vi "Read Logger.vi"(8 "error in (no error)":errorcluster, 11 "CoreOperation in":refnum<class "CoreOperation.lvclass">) -> (0 "error out":errorcluster, 2 "Logger.lvclass":refnum<class "Logger.lvclass">, 3 "CoreOperation out":refnum<class "CoreOperation.lvclass">)   [LabVIEW 2014, in "CoreOperation.lvclass"]
uses:
  CoreOperation.lvclass
  Utilities/Logger/Logger.lvclass
  CoreOperation.lvclass/CoreOperation.ctl
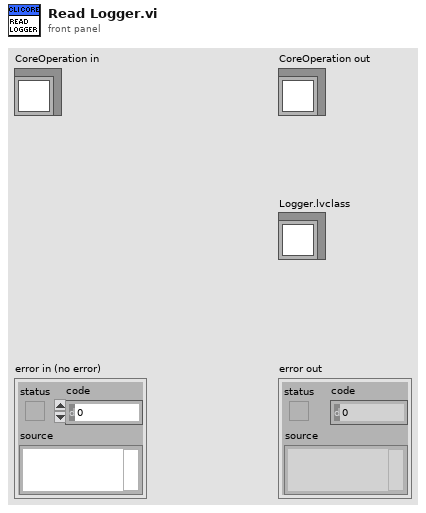
[diagram p1: front panel]
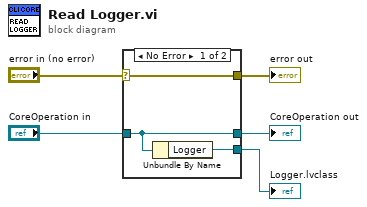
[diagram p0: block diagram]
diagram:
  n1 = case shown="No Error" "error in (no error)" {
    selector: "error in (no error)" -> [w8 w9]
    tunnel: [w8 w9] -> w4
    tunnel: [w7 w10] -> w2
    tunnel: "CoreOperation in" -> [w7 w10]
    tunnel: [w6 _] -> w1
    frame No Error {
      n2 = Unbundle By Name(w7) -> ("Logger"=w6:refnum<class "Logger.lvclass">)
    }
    frame Error {
    }
  }
  "error out" <- w4
  "CoreOperation out" <- w2
  "Logger.lvclass" <- w1
